vi "Update.vi"(4 "Value2":dbl, 6 "Value1":dbl, 8 "error in (no error)":errorcluster, 9 "Audio History Buffer In":dbl[][](array[numeric]), 10 "Audio Data In":dbl[][](array[numeric]), 11 "Echo in":refnum<class "Echo.lvclass">) -> (0 "error out":errorcluster, 1 "Audio History Buffer Out":dbl[][](array[numeric]), 2 "Audio Data Out":dbl[][](array[numeric]), 3 "Echo out":refnum<class "Echo.lvclass">)   [LabVIEW 2018, in "Echo.lvlib" / "Echo.lvclass"]
doc: "Applies an echo effect to the audio. A delayed copy of the audio signal is added to the original signal. The resulting signal is output, but also stored in <b>Audio History Buffer Out</b> for reuse in subsequent iterations.\n\n<b>Value1:</b> Feedback amount\n<b>Value2:</b> Echo delay"
uses:
  Echo.lvclass
  Libraries/Globals/Constants.vi
  Libraries/Globals/Globals.lvlib
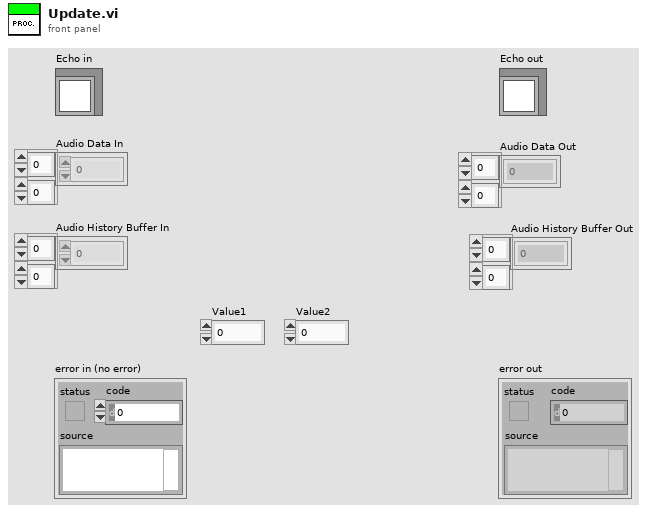
[diagram p1: front panel]
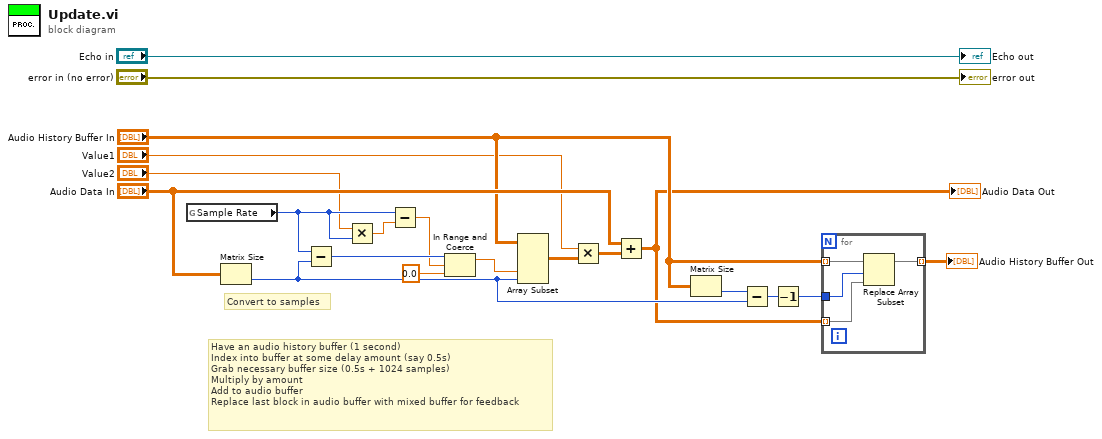
[diagram p0: block diagram]
diagram:
  # "Convert to samples"
  # "Have an audio history buffer (1 second)\nIndex into buffer at some delay amount (say 0.5s)\nGrab necessary buffer size (0.5s + 1024 samples)\nMultiply by amount\nAdd to audio buffer\nReplace last block in audio buffer with mixed buffer for feedback"
  n1 = global read "Constants.vi" "Sample Rate"() -> (w7:i32)
  n2 = Matrix Size(0:"Audio Data In") -> (2:w12:i32)  [unwired: 1 out]
  n3 = Subtract(x=w7, y=w12) -> (x-y=w11:i32)
  n4 = Multiply(x="Value2", y=w7) -> (x*y=w18:dbl)
  n5 = Subtract(x=w7, y=w18) -> (x-y=w10:dbl)
  n6 = In Range and Coerce(upper limit=w11, x=w10, lower limit=0.0) -> (coerced(x)=w8:dbl)  [unwired: 1 out]
  n7 = Array Subset(array="Audio History Buffer In", index (col)=w8, length (col)=w12) -> (w17:dbl[][])  [unwired: 2 in]
  n8 = Multiply(x="Value1", y=w17) -> (x*y=w16:dbl[][])
  n9 = Add(x="Audio Data In", y=w16) -> (x+y=w4:dbl[][])
  "Audio Data Out" <- w4
  n10 = Matrix Size(0:"Audio History Buffer In") -> (2:w15:i32)  [unwired: 1 out]
  n11 = Subtract(x=w15, y=w12) -> (x-y=w14:i32)
  n12 = Decrement(x=w14) -> (x-1=w13:i32)
  n13 = for {
    tunnel: w13 -> [w23]
    tunnel: "Audio History Buffer In" -> [w24] mode=indexing
    tunnel: [w22] -> w3 mode=indexing
    tunnel: w4 -> [w21] mode=indexing
    n14 = Replace Array Subset(array=w24, new element=w21, index=w23) -> (w22:dbl[])
  }
  "Audio History Buffer Out" <- w3
  "error out" <- "error in (no error)"
  "Echo out" <- "Echo in"
